vi "Arm State Controller v2.vi"(0 "Elbow Manual Power":dbl, 1 "Shoulder Manual Power":dbl, 2 "Setpoint Change Detected?":bool, 3 "Target Arm State":T1(ring)) -> ()   [LabVIEW 2020]
uses:
  <vilib>/Rock Robotics/WPI/ThirdParty/REV Robotics/REVLib/Typedef/Spark MAX Control Type.ctl
  Robot Global Data.vi
panel:
  in  "Target Shoulder":dbl
  in  "Target Elbow":dbl
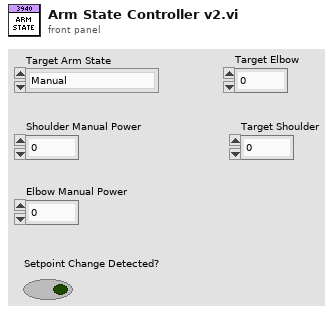
[diagram p1: front panel]
types:
  T1 = enum16{"Manual", "High Cone", "High Cube", "Mid Cone", "Mid Cube", "Intake", "Cube Handoff", "Cone Handoff", "Stow"}
  T2 = cluster{"Stow Elbow Setpoint":dbl, "Intake Elbow Setpoint":dbl, "Cube Handoff Elbow Setpoint":dbl, "Cone Handoff Elbow Setpoint":dbl, "Mid Cone Elbow Setpoint":dbl, "Mid Cube Elbow Setpoint":dbl, "High Cone Elbow Setpoint":dbl, "High Cube Elbow Setpoint":dbl}
  T3 = cluster{"Stow Shoulder Setpoint":dbl, "Intake Shoulder Setpoint":dbl, "Cube Handoff Shoulder Setpoint":dbl, "Cone Handoff Shoulder Setpoint":dbl, "Mid Cone Shoulder Setpoint":dbl, "Mid Cube Shoulder Setpoint":dbl, "High Cone Shoulder Setpoint":dbl, "High Cube Shoulder Setpoint":dbl}
  T4 = typedef "WPI_MotorControlDeviceRef.ctl" = cluster{"DeviceStatus":errorcluster, "Type":T5, "PWM":cluster{"PWM Channel":T6, "DeadBand":T7}, "CAN":cluster{"Device Number":u8, "SetOutput VI Ref":variant, "GetOutput VI Ref":variant, "Enable VI Ref":variant, "Disable VI Ref":variant, "Data":variant}, "Invert":bool, "DIO PWM":cluster{"PWM \"Enable\" Channel":T6, "DIOChannel":T8, "PWM Rate":dbl}}
  T5 = typedef "WPI_MotorControlType.ctl" = enum16{"PWM", "CAN", "DIO PWM"}
  T6 = typedef "FPGA_DIOPWMChannel.ctl" = enum8{"PWM 0", "PWM 1", "PWM 2", "PWM 3", "PWM 4", "PWM 5", "PWM 6", "PWM 7", "PWM 8", "PWM 9", "PWM MXP 0", "PWM MXP 1", "PWM MXP 2", "PWM MXP 3", "PWM MXP 4", "PWM MXP 5", "PWM MXP 6", "PWM MXP 7", "PWM MXP 8", "PWM MXP 9", "Invalid"}
  T7 = typedef "WPI_PWMDeadband.ctl" = cluster{"Name":string, "maxPositivePwm":i32, "minPositivePwm":i32, "centerPwm":i32, "maxNegativePwm":i32, "minNegativePwm":i32, "angularRange":u16}
  T8 = typedef "FPGA_DIOChannel.ctl" = enum8{"DIO 0", "DIO 1", "DIO 2", "DIO 3", "DIO 4", "DIO 5", "DIO 6", "DIO 7", "DIO 8", "DIO 9", "DIO MXP 0", "DIO MXP 1", "DIO MXP 2", "DIO MXP 3", "DIO MXP 4", "DIO MXP 5", "DIO MXP 6", "DIO MXP 7", "DIO MXP 8", "DIO MXP 9", "DIO MXP 10", "DIO MXP 11", "DIO MXP 12", "DIO MXP 13", "DIO MXP 14", "DIO MXP 15", "SPI Port CS1", "SPI Port CS2", "SPI Port CS3", "SPI Port MISO", "SPI Port MOSI", "Invalid"}
  T9 = typedef "Spark MAX Control Type.ctl" = enum16{"Percent VBus", "Voltage", "Velocity", "Position", "Smart Motion", "Current", "Smart Velocity"}
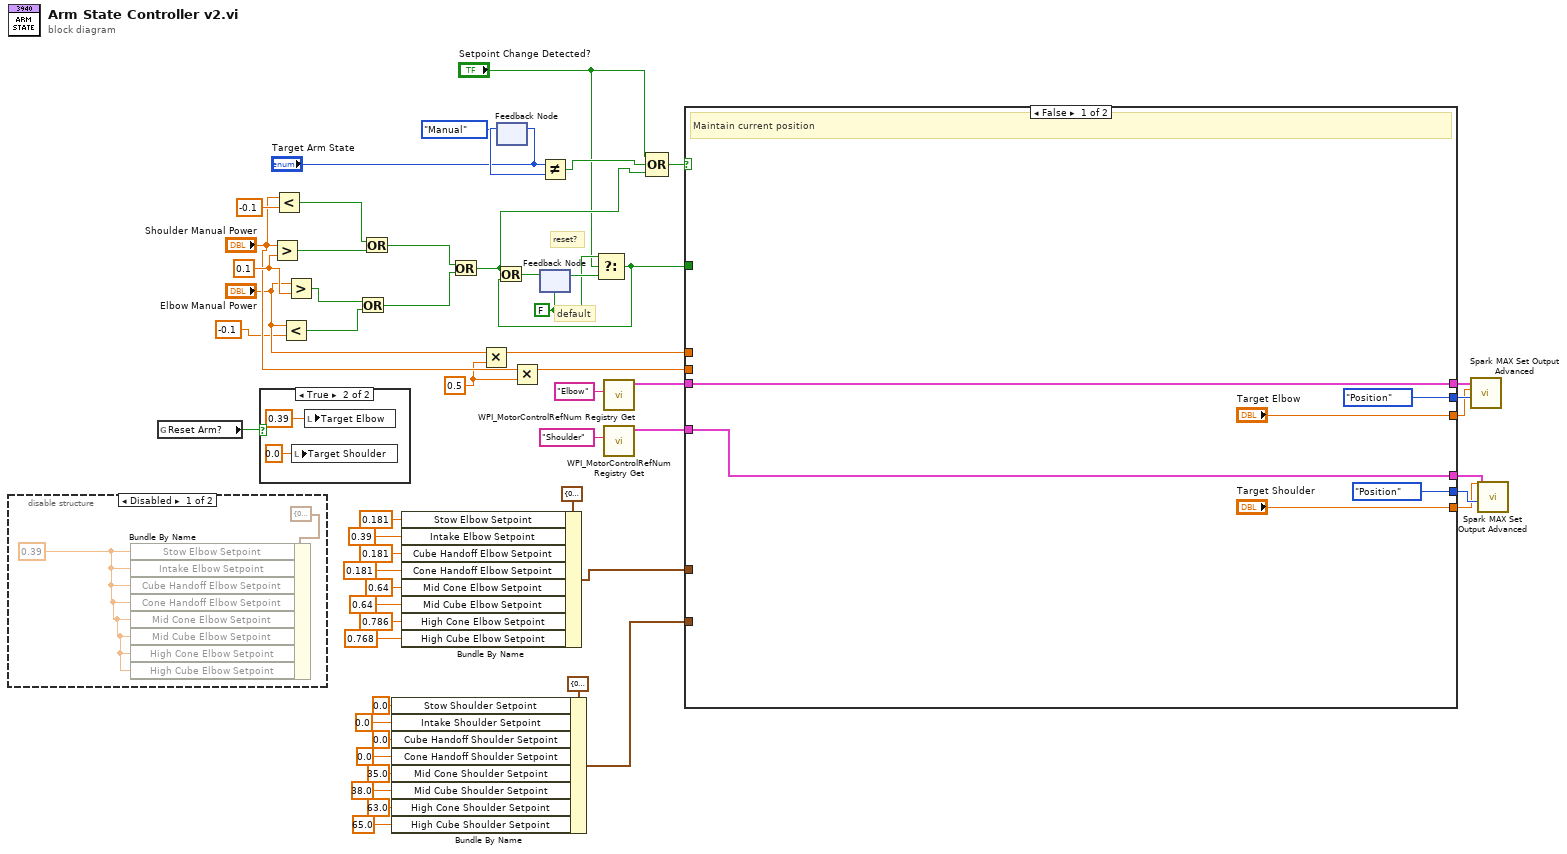
[diagram p0: block diagram]
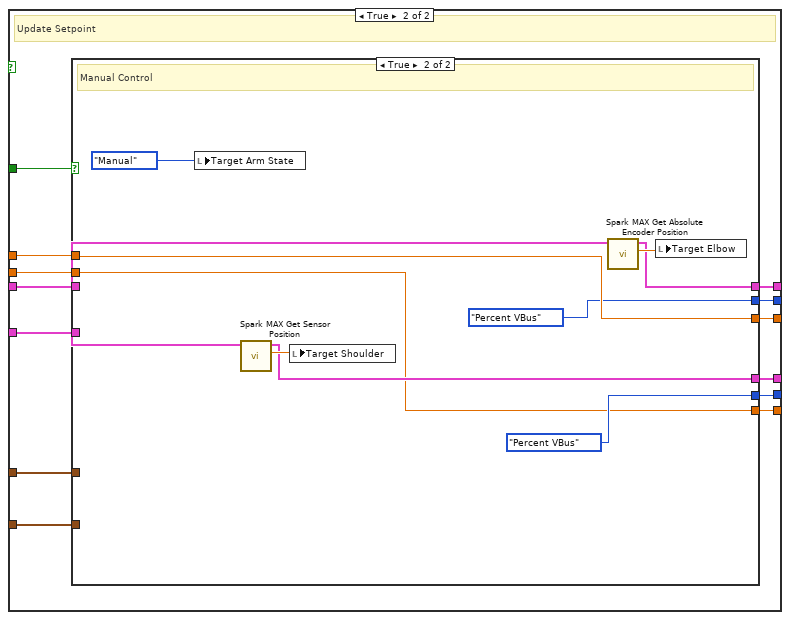
[diagram p4: hidden frame]
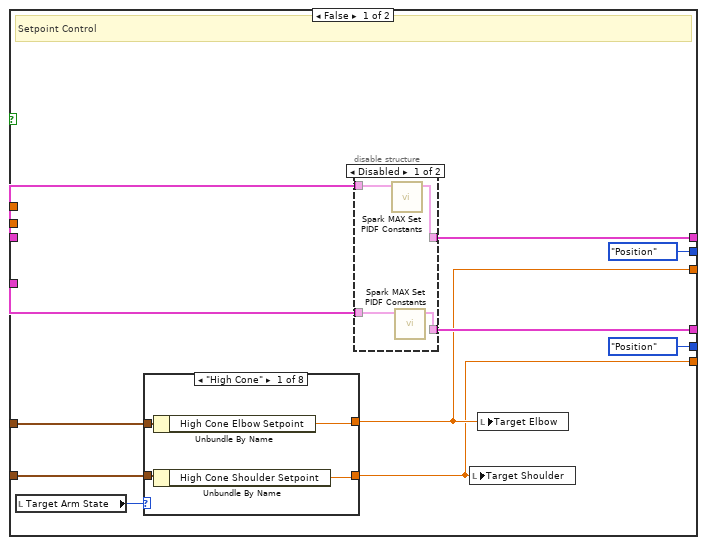
[diagram p5: hidden frame]
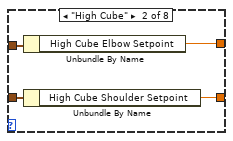
[diagram p7: hidden frame]
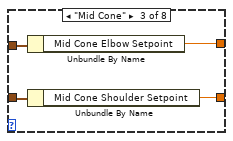
[diagram p8: hidden frame]
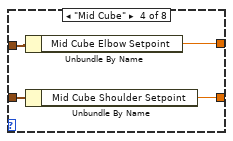
[diagram p9: hidden frame]
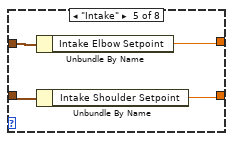
[diagram p10: hidden frame]
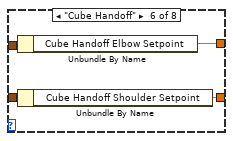
[diagram p11: hidden frame]
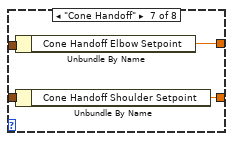
[diagram p12: hidden frame]
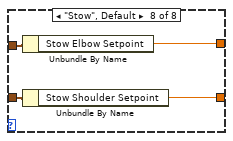
[diagram p13: hidden frame]
diagram:
  w11 = 0.5 ("y")
  w45 = FALSE
  w35 = 0.1 ("y")
  # "default"
  # "reset?"
  n1 = disable-structure shown="Disabled" {
    frame Disabled {
      w58 = 0.39 ("Stow Elbow Setpoint")
      n2 = Bundle By Name(cluster=T2 {"Stow Elbow Setpoint"=0.0, "Intake Elbow Setpoint"=0.0, "Cube Handoff Elbow Setpoint"=0.0, "Cone Handoff Elbow Setpoint"=0.0, "Mid Cone Elbow Setpoint"=0.0, "Mid Cube Elbow Setpoint"=0.0, "High Cone Elbow Setpoint"=0.0, "High Cube Elbow Setpoint"=0.0}, "Stow Elbow Setpoint"=w58, "Intake Elbow Setpoint"=w58, "Cube Handoff Elbow Setpoint"=w58, "Cone Handoff Elbow Setpoint"=w58, "Mid Cone Elbow Setpoint"=w58, "Mid Cube Elbow Setpoint"=w58, "High Cone Elbow Setpoint"=w58, "High Cube Elbow Setpoint"=w58) -> ()  [unwired: 1 out]
    }
    frame Enabled {
    }
  }
  n3 = global read "Robot Global Data.vi" "Reset Arm?"() -> (w14:bool)
  n4 = case shown="True" w14 {
    frame False {
    }
    frame True {
      n5 = local write "Target Shoulder"(0.0 ("Target Shoulder")) -> ()
      n6 = local write "Target Elbow"(0.39 ("Target Elbow")) -> ()
    }
  }
  n7 = Greater?(x="Shoulder Manual Power", y=w35) -> (0:w38:bool)
  n8 = Less?(x="Shoulder Manual Power", y=-0.1) -> (x < y?=w37:bool)
  n9 = Less?(x="Elbow Manual Power", y=-0.1 ("x")) -> (x < y?=w30:bool)
  n10 = Greater?(x="Elbow Manual Power", y=w35) -> (0:w31:bool)
  n11 = Or(x=w31, y=w30) -> (x .or. y?=w29:bool)
  n12 = Or(x=w37, y=w38) -> (x .or. y?=w28:bool)
  n13 = Bundle By Name(cluster=T3 {"Stow Shoulder Setpoint"=0.0, "Intake Shoulder Setpoint"=0.0, "Cube Handoff Shoulder Setpoint"=0.0, "Cone Handoff Shoulder Setpoint"=0.0, "Mid Cone Shoulder Setpoint"=0.0, "Mid Cube Shoulder Setpoint"=0.0, "High Cone Shoulder Setpoint"=0.0, "High Cube Shoulder Setpoint"=0.0}, "Stow Shoulder Setpoint"=0.0 ("Stow Elbow Setpoint"), "Intake Shoulder Setpoint"=0.0 ("Intake Elbow Setpoint"), "Cube Handoff Shoulder Setpoint"=0.0 ("Cube Handoff Elbow Setpoint"), "Cone Handoff Shoulder Setpoint"=0.0 ("Cone Handoff Elbow Setpoint"), "Mid Cone Shoulder Setpoint"=35.0 ("Mid Cone Elbow Setpoint"), "Mid Cube Shoulder Setpoint"=38.0 ("Mid Cube Elbow Setpoint"), "High Cone Shoulder Setpoint"=63.0 ("High Cone Elbow Setpoint"), "High Cube Shoulder Setpoint"=65.0 ("High Cube Elbow Setpoint")) -> (w39:T3)
  n14 = Bundle By Name(cluster=T2 {"Stow Elbow Setpoint"=0.0, "Intake Elbow Setpoint"=0.0, "Cube Handoff Elbow Setpoint"=0.0, "Cone Handoff Elbow Setpoint"=0.0, "Mid Cone Elbow Setpoint"=0.0, "Mid Cube Elbow Setpoint"=0.0, "High Cone Elbow Setpoint"=0.0, "High Cube Elbow Setpoint"=0.0}, "Stow Elbow Setpoint"=0.181, "Intake Elbow Setpoint"=0.39, "Cube Handoff Elbow Setpoint"=0.181, "Cone Handoff Elbow Setpoint"=0.181, "Mid Cone Elbow Setpoint"=0.64, "Mid Cube Elbow Setpoint"=0.64, "High Cone Elbow Setpoint"=0.786, "High Cube Elbow Setpoint"=0.768) -> (w1:T2)
  n15 = Or(x=w28, y=w29) -> (x .or. y?=w17:bool)
  n16 = Multiply(x="Elbow Manual Power", y=w11) -> (x*y=w13:dbl)
  n17 = feedback-in #1("Target Arm State") -> ()
  n18 = feedback #1(T1."Manual" ("Target Arm State")) -> (w27:T1)
  n19 = Multiply(x="Shoulder Manual Power", y=w11) -> (x*y=w12:dbl)
  n20 = Not Equal?(x="Target Arm State", y=w27) -> (x != y?=w18:bool)
  n21 = feedback #2(w45) -> (w46:bool)
  n22 = Select(t=w45, s="Setpoint Change Detected?", f=w46) -> (s? t:f=w44:bool)
  n23 = Or(x=w17, y=w44) -> (x .or. y?=w47:bool)
  n24 = feedback-in #2(w47) -> ()
  n25 = call <vilib>:"WPI_MotorControlRefNum Registry Get.vi"("refnum name"="Elbow") -> ("MotorControlDevRef"=w41:T4)  [unwired: 9 in, 1 out]
  n26 = call <vilib>:"WPI_MotorControlRefNum Registry Get.vi"("refnum name"="Shoulder") -> ("MotorControlDevRef"=w40:T4)  [unwired: 9 in, 1 out]
  n27 = Compound Arithmetic op=OR("Setpoint Change Detected?", w18, w17) -> (w16:bool)
  n28 = case shown="False" w16 {
    tunnel: w44 -> [_ w79]
    tunnel: w13 -> [_ w78]
    tunnel: w12 -> [_ w77]
    tunnel: w41 -> [w65 w76]
    tunnel: w40 -> [w61 w75]
    tunnel: w1 -> [_ w74]
    tunnel: w39 -> [_ w73]
    tunnel: [Spark_MAX_Control_Type."Position" ("Control Mode") w71] -> w24
    tunnel: [w65 w70] -> w23
    tunnel: ["Target Elbow" w68] -> w22
    tunnel: [Spark_MAX_Control_Type."Position" ("Control Mode") w72] -> w21
    tunnel: ["Target Shoulder" w67] -> w20
    tunnel: [w61 w69] -> w19
    frame False {
      # "Maintain current position"
    }
    frame True {
      # "Update Setpoint"
      n29 = case shown="True" w79 {
        tunnel: w78 -> [_ w135]
        tunnel: w77 -> [_ w128]
        tunnel: w76 -> [w90 w134]
        tunnel: w75 -> [w89 w131]
        tunnel: w74 -> [w87 _]
        tunnel: w73 -> [w86 _]
        tunnel: [Spark_MAX_Control_Type."Position" ("Control Mode") Spark_MAX_Control_Type."Percent VBus" ("Control Mode")] -> w72
        tunnel: [Spark_MAX_Control_Type."Position" ("Control Mode") Spark_MAX_Control_Type."Percent VBus" ("Control Mode")] -> w71
        tunnel: [w83 w133] -> w70
        tunnel: [w82 w130] -> w69
        tunnel: [w81 w135] -> w68
        tunnel: [w80 w128] -> w67
        frame False {
          # "Setpoint Control"
          n30 = local read "Target Arm State"() -> (w88:T1)
          n31 = case shown="\"High Cone\"" w88 {
            tunnel: w87 -> [w98 w102 w106 w110 w114 w118 w122 w126]
            tunnel: w86 -> [w97 w101 w105 w109 w113 w117 w120 w125]
            tunnel: [w96 w100 w104 w108 w112 w116 w121 w124] -> w81
            tunnel: [w95 w99 w103 w107 w111 w115 w119 w123] -> w80
            frame "High Cone" {
              n32 = Unbundle By Name(w98) -> ("High Cone Elbow Setpoint"=w96:dbl)
              n33 = Unbundle By Name(w97) -> ("High Cone Shoulder Setpoint"=w95:dbl)
            }
            frame "High Cube" {
              n34 = Unbundle By Name(w102) -> ("High Cube Elbow Setpoint"=w100:dbl)
              n35 = Unbundle By Name(w101) -> ("High Cube Shoulder Setpoint"=w99:dbl)
            }
            frame "Mid Cone" {
              n36 = Unbundle By Name(w106) -> ("Mid Cone Elbow Setpoint"=w104:dbl)
              n37 = Unbundle By Name(w105) -> ("Mid Cone Shoulder Setpoint"=w103:dbl)
            }
            frame "Mid Cube" {
              n38 = Unbundle By Name(w110) -> ("Mid Cube Elbow Setpoint"=w108:dbl)
              n39 = Unbundle By Name(w109) -> ("Mid Cube Shoulder Setpoint"=w107:dbl)
            }
            frame "Intake" {
              n40 = Unbundle By Name(w114) -> ("Intake Elbow Setpoint"=w112:dbl)
              n41 = Unbundle By Name(w113) -> ("Intake Shoulder Setpoint"=w111:dbl)
            }
            frame "Cube Handoff" {
              n42 = Unbundle By Name(w118) -> ("Cube Handoff Elbow Setpoint"=w116:dbl)
              n43 = Unbundle By Name(w117) -> ("Cube Handoff Shoulder Setpoint"=w115:dbl)
            }
            frame "Cone Handoff" {
              n44 = Unbundle By Name(w122) -> ("Cone Handoff Elbow Setpoint"=w121:dbl)
              n45 = Unbundle By Name(w120) -> ("Cone Handoff Shoulder Setpoint"=w119:dbl)
            }
            frame "Stow", Default {
              n46 = Unbundle By Name(w126) -> ("Stow Elbow Setpoint"=w124:dbl)
              n47 = Unbundle By Name(w125) -> ("Stow Shoulder Setpoint"=w123:dbl)
            }
          }
          n48 = disable-structure shown="Disabled" {
            disable-tunnel: w90 -> [w94 _]
            disable-tunnel: w89 -> [w93 _]
            disable-tunnel: [w92 _] -> w83
            disable-tunnel: [w91 _] -> w82
            frame Disabled {
              n49 = call <vilib>:"Spark MAX Set PIDF Constants.vi"("MotorControlDeviceRef"=w94) -> ("MotorControlDeviceRef"=w92:T4)  [unwired: 9 in, 1 out]
              n50 = call <vilib>:"Spark MAX Set PIDF Constants.vi"("MotorControlDeviceRef"=w93) -> ("MotorControlDeviceRef"=w91:T4)  [unwired: 9 in, 1 out]
            }
            frame Enabled {
            }
          }
          n51 = local write "Target Shoulder"(w80) -> ()
          n52 = local write "Target Elbow"(w81) -> ()
        }
        frame True {
          # "Manual Control"
          n53 = local write "Target Arm State"(T1."Manual" ("Target Arm State")) -> ()
          n54 = call <vilib>:"Spark MAX Get Sensor Position.vi"("MotorControlDevRef in"=w131) -> ("Sensor Position"=w136:dbl, "MotorControlDevRef out"=w130:T4)  [unwired: 7 in, 2 out]
          n55 = local write "Target Shoulder"(w136) -> ()
          n56 = call <vilib>:"Spark MAX Get Absolute Encoder Position.vi"("MotorControlDeviceRef in"=w134) -> ("Position"=w137:dbl, "MotorControlDeviceRef out"=w133:T4)  [unwired: 7 in, 2 out]
          n57 = local write "Target Elbow"(w137) -> ()
        }
      }
    }
  }
  n58 = call <vilib>:"Spark MAX Set Output Advanced.vi"("Control Mode"=w24, "Setpoint"=w22, "MotorControlDevRef"=w23) -> ()  [unwired: 7 in, 2 out]
  n59 = call <vilib>:"Spark MAX Set Output Advanced.vi"("Control Mode"=w21, "Setpoint"=w20, "MotorControlDevRef"=w19) -> ()  [unwired: 7 in, 2 out]
